vi "DEMO.vi"() -> ()   [LabVIEW 2013]
uses:
  Data.lvclass/DataControlType.ctl
  Data.lvclass/Data.lvclass
panel:
  in  "ICP":bool
  in  "ACCoupling":bool
  in  "ChannelAliasName":string
  in  "PhysicalChannel":string
  in  "Sample#":dbl
  in  "Rate":dbl
  out "Cluster Out":T1
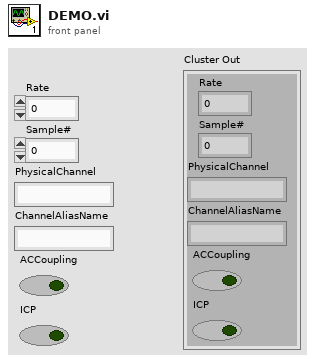
[diagram p1: front panel]
types:
  T1 = typedef "Data.lvclass/DataControlType.ctl" = cluster{"Rate":dbl, "Sample#":dbl, "PhysicalChannel":string, "ChannelAliasName":string, "ACCoupling":bool, "ICP":bool}
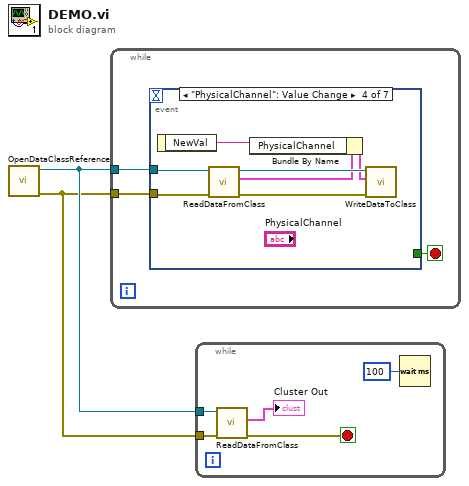
[diagram p0: block diagram]
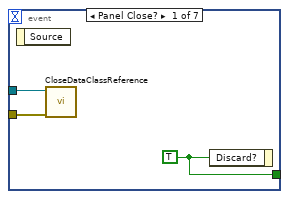
[diagram p2: hidden frame]
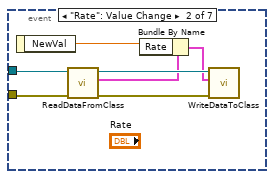
[diagram p3: hidden frame]
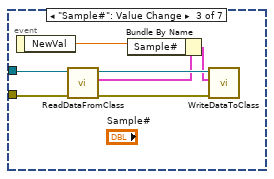
[diagram p4: hidden frame]
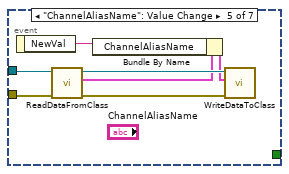
[diagram p5: hidden frame]
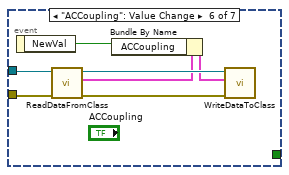
[diagram p6: hidden frame]
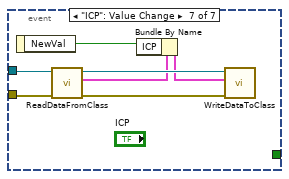
[diagram p7: hidden frame]
diagram:
  n1 = call "OpenDataClassReference.vi"() -> ("error out"=w1:errorcluster, "DataClassNotifier out"=w2:refnum<notifier>)  [unwired: 10 in]
  n2 = while {
    tunnel: w1 -> [w3]
    tunnel: w2 -> [w4]
    stop <- w5 stop-if-true
    n3 = event shown="[3] \"PhysicalChannel\": Value Change" {
      selector: _ -> [_ _ _ _ _ _ _]
      dyn-events: _ -> [_ _ _ _ _ _ _]
      timeout: _ -> [_ _ _ _ _ _ _]
      tunnel: [w8 _ _ _ _ _ _] -> w5
      tunnel: w4 -> [w7 w15 w22 w29 w36 w43 w50]
      tunnel: w3 -> [w6 w12 w19 w26 w33 w40 w47]
      event Panel Close? {
        w8 = TRUE ("Discard?")
        n4 = event-data() -> ()  [unwired: 1 in, 1 out]
        n5 = call "CloseDataClassReference.vi"("error in (no error)"=w6, "DataClassNotifierIn"=w7) -> ()  [unwired: 8 in, 2 out]
        n6 = event-data("Discard?"=w8) -> ()  [unwired: 1 in, 1 out]
      }
      event "Rate": Value Change {
        n7 = event-data() -> ("NewVal"=w9:dbl)  [unwired: 1 in]
        n8 = call "ReadDataFromClass.vi"("error in (no error)"=w12, "DataClassNotifierIn"=w15) -> ("error out"=w13:errorcluster, "Cluster"=w11:T1, "DataClassNotifierOut"=w14:refnum<notifier>)  [unwired: 7 in]
        n9 = Bundle By Name(cluster=w11, "Rate"=w9) -> (w10:T1)
        n10 = call "WriteDataToClass.vi"("error in (no error)"=w13, "Cluster"=w10, "DataClassNotifier out"=w14) -> ()  [unwired: 7 in, 2 out]
      }
      event "Sample#": Value Change {
        n11 = event-data() -> ("NewVal"=w16:dbl)  [unwired: 1 in]
        n12 = call "ReadDataFromClass.vi"("error in (no error)"=w19, "DataClassNotifierIn"=w22) -> ("error out"=w20:errorcluster, "Cluster"=w18:T1, "DataClassNotifierOut"=w21:refnum<notifier>)  [unwired: 7 in]
        n13 = Bundle By Name(cluster=w18, "Sample#"=w16) -> (w17:T1)
        n14 = call "WriteDataToClass.vi"("error in (no error)"=w20, "Cluster"=w17, "DataClassNotifier out"=w21) -> ()  [unwired: 7 in, 2 out]
      }
      event "PhysicalChannel": Value Change {
        n15 = event-data() -> ("NewVal"=w23:string)  [unwired: 1 in]
        n16 = call "ReadDataFromClass.vi"("error in (no error)"=w26, "DataClassNotifierIn"=w29) -> ("error out"=w27:errorcluster, "Cluster"=w25:T1, "DataClassNotifierOut"=w28:refnum<notifier>)  [unwired: 7 in]
        n17 = Bundle By Name(cluster=w25, "PhysicalChannel"=w23) -> (w24:T1)
        n18 = call "WriteDataToClass.vi"("error in (no error)"=w27, "Cluster"=w24, "DataClassNotifier out"=w28) -> ()  [unwired: 7 in, 2 out]
      }
      event "ChannelAliasName": Value Change {
        n19 = event-data() -> ("NewVal"=w30:string)  [unwired: 1 in]
        n20 = call "ReadDataFromClass.vi"("error in (no error)"=w33, "DataClassNotifierIn"=w36) -> ("error out"=w34:errorcluster, "Cluster"=w32:T1, "DataClassNotifierOut"=w35:refnum<notifier>)  [unwired: 7 in]
        n21 = Bundle By Name(cluster=w32, "ChannelAliasName"=w30) -> (w31:T1)
        n22 = call "WriteDataToClass.vi"("error in (no error)"=w34, "Cluster"=w31, "DataClassNotifier out"=w35) -> ()  [unwired: 7 in, 2 out]
      }
      event "ACCoupling": Value Change {
        n23 = event-data() -> ("NewVal"=w37:bool)  [unwired: 1 in]
        n24 = call "ReadDataFromClass.vi"("error in (no error)"=w40, "DataClassNotifierIn"=w43) -> ("error out"=w41:errorcluster, "Cluster"=w39:T1, "DataClassNotifierOut"=w42:refnum<notifier>)  [unwired: 7 in]
        n25 = Bundle By Name(cluster=w39, "ACCoupling"=w37) -> (w38:T1)
        n26 = call "WriteDataToClass.vi"("error in (no error)"=w41, "Cluster"=w38, "DataClassNotifier out"=w42) -> ()  [unwired: 7 in, 2 out]
      }
      event "ICP": Value Change {
        n27 = event-data() -> ("NewVal"=w44:bool)  [unwired: 1 in]
        n28 = call "ReadDataFromClass.vi"("error in (no error)"=w47, "DataClassNotifierIn"=w50) -> ("error out"=w48:errorcluster, "Cluster"=w46:T1, "DataClassNotifierOut"=w49:refnum<notifier>)  [unwired: 7 in]
        n29 = Bundle By Name(cluster=w46, "ICP"=w44) -> (w45:T1)
        n30 = call "WriteDataToClass.vi"("error in (no error)"=w48, "Cluster"=w45, "DataClassNotifier out"=w49) -> ()  [unwired: 7 in, 2 out]
      }
    }
  }
  n31 = while {
    tunnel: w2 -> [w54]
    tunnel: w1 -> [w53]
    stop <- w52 stop-if-true
    n32 = call "ReadDataFromClass.vi"("error in (no error)"=w53, "DataClassNotifierIn"=w54) -> ("error out"=w52:errorcluster, "Cluster"=→"Cluster Out":T1)  [unwired: 7 in, 1 out]
    n33 = Wait (ms)(milliseconds to wait=u32 100) -> ()  [unwired: 1 out]
  }
